vi "Averaging.vi"(8 "old input array":dbl[][](array[numeric]), 9 "new input array":dbl[][](array[numeric]), 10 "Number of averages":i32, 11 "current measurement number":i32) -> (0 "output array":dbl[][](array[numeric]), 3 "next measurement number":i32)   [LabVIEW 2013]
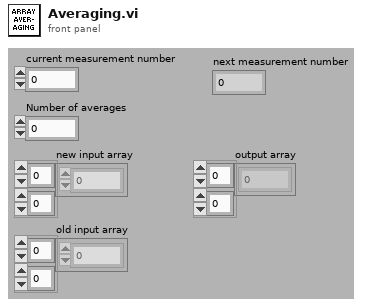
[diagram p1: front panel]
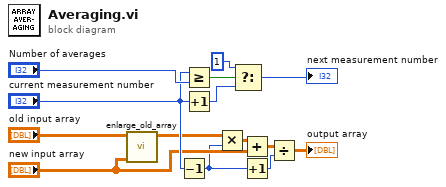
[diagram p0: block diagram]
diagram:
  n1 = call "enlarge_old_array.vi"("new input array"="new input array", "old input array (IN)"="old input array") -> ("old input array (OUT)"=w1:dbl[][])  [unwired: 9 in]
  n2 = Decrement(x="current measurement number") -> (x-1=w2:i32)
  n3 = Greater Or Equal?(x="current measurement number", y="Number of averages") -> (x >= y?=w5:bool)
  n4 = Increment(x="current measurement number") -> (x+1=w6:i32)
  n5 = Multiply(x=w1, y=w2) -> (x*y=w8:dbl[][])
  n6 = Select(t=1, s=w5, f=w6) -> (s? t:f=→"next measurement number":i32)
  n7 = Add(x=w8, y="new input array") -> (x+y=w7:dbl[][])
  n8 = Increment(x=w2) -> (x+1=w4:i32)
  n9 = Divide(x=w7, y=w4) -> (x/y=→"output array":dbl[][])
